vi "Rio_Theta_Movement_Main (DONE).vi"(7 "Desired Position":dbl step=0.9, 8 "Error In":errorcluster) -> (0 "error out":errorcluster)   [LabVIEW 2017]
doc: "This VI calibrates the Theta axis to is \"home\" position before moving it to the desired input angle/position.\n\nWritten by Stefan Clarkson, Robin Moore & Thomas Quinn 26/02/18."
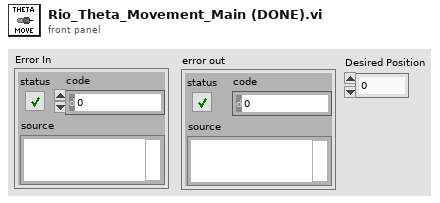
[diagram p1: front panel]
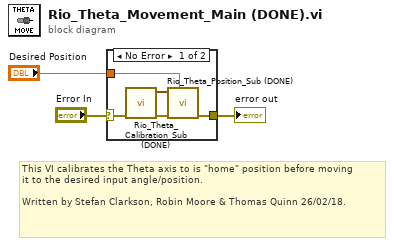
[diagram p0: block diagram]
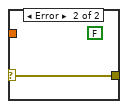
[diagram p2: hidden frame]
diagram:
  # "This VI calibrates the Theta axis to is \"home\" position before moving \nit to the desired input angle/position.\n\nWritten by Stefan Clarkson, Robin Moore & Thomas Quinn 26/02/18."
  n1 = case shown="No Error" "Error In" {
    selector: "Error In" -> [w6 w9]
    tunnel: [w8 w9] -> w2
    tunnel: "Desired Position" -> [w4 _]
    frame No Error {
      n2 = call "Rio_Theta_Calibration_Sub (DONE).vi"("error in (no error)"=w6) -> ("error out"=w7:errorcluster, "Theta Sequence & Position"=w5:cluster{i32, dbl})  [unwired: 9 in]
      n3 = call "Rio_Theta_Position_Sub (DONE).vi"("Desired Position"=w4, "error in (no error)"=w7, "Theta Sequence & Position"=w5) -> ("error out"=w8:errorcluster)  [unwired: 8 in]
    }
    frame Error {
      (unwired) FALSE ("Movement Complete")
    }
  }
  "error out" <- w2
